vi "getInstance.vi"(8 "error in (no error)":errorcluster) -> (0 "error out":errorcluster, 3 "Instance out":refnum<data-value>)   [LabVIEW 2017, in "SingleObject.lvclass"]
uses:
  SingleObject.lvclass
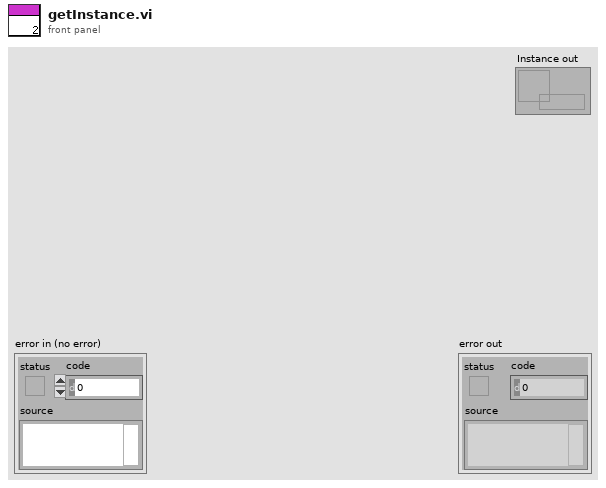
[diagram p1: front panel]
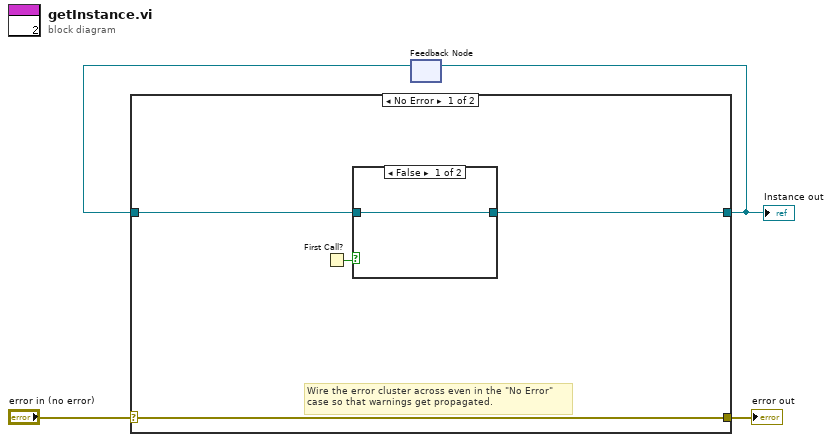
[diagram p0: block diagram]
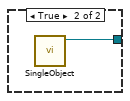
[diagram p2: hidden frame]
diagram:
  n1 = feedback #1() -> (w1:refnum<data-value>)  [unwired: 1 in]
  n2 = case shown="No Error" "error in (no error)" {
    selector: "error in (no error)" -> [w8 w12]
    tunnel: [w8 w12] -> w3
    tunnel: [w7 w11] -> w2
    tunnel: w1 -> [w5 w11]
    frame No Error {
      # "Wire the error cluster across even in the \"No Error\"\ncase so that warnings get propagated."
      n3 = First Call?() -> (First Call?: T/F=w6:bool)
      n4 = case shown="False" w6 {
        tunnel: [w9 w10] -> w7
        tunnel: w5 -> [w9 _]
        frame False {
        }
        frame True {
          n5 = call "SingleObject.vi"() -> ("Instance out"=w10:refnum<data-value>)  [unwired: 10 in, 1 out]
        }
      }
    }
    frame Error {
    }
  }
  "error out" <- w3
  "Instance out" <- w2
  n6 = feedback-in #1(w2) -> ()
